vi "Set Conditional Symbols.vi"(0 "Project Path":path, 1 "w_niscope":bool, 2 "w_visa":bool, 11 "error in (no error)":errorcluster) -> (15 "error out":errorcluster)   [LabVIEW 2013]
doc: "VI sets conditional symbols in the project."
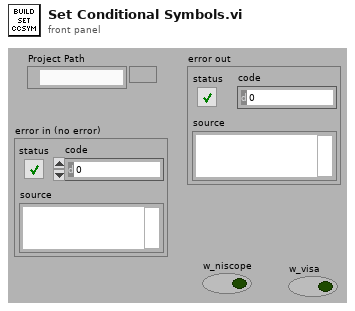
[diagram p1: front panel]
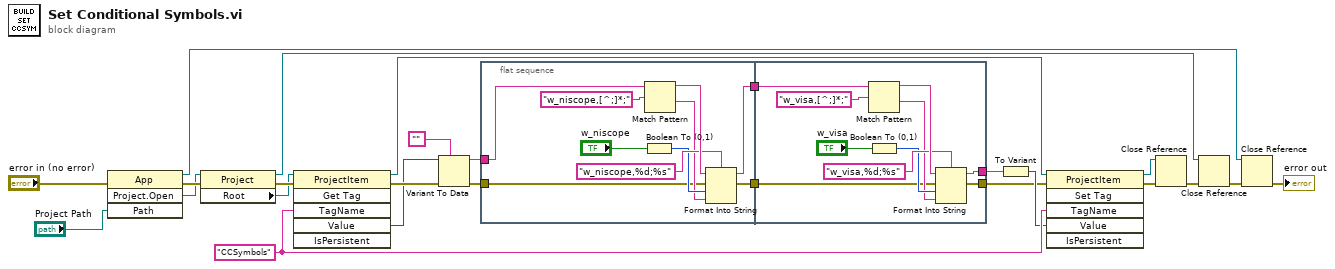
[diagram p0: block diagram]
diagram:
  w22 = "CCSymbols" ("Tag Name")
  n1 = invoke class="App" method="Project.Open"(error in="error in (no error)", "Path"="Project Path") -> (reference out=w13:refnum<vi>, error out=w14:errorcluster, "Project:Open"=w11:refnum<vi>)  [unwired: 2 in, 1 out]
  n2 = property class="Project"(reference=w11, error in=w14) -> (reference out=w12:refnum<vi>, error out=w21:errorcluster, "Root"=w2:refnum<vi>)
  n3 = invoke class="ProjectItem" method="Get Tag"(reference=w2, error in=w21, "TagName"=w22) -> (reference out=w1:refnum<vi>, error out=w24:errorcluster, "Value"=w23:variant)  [unwired: 3 in, 3 out]
  n4 = Variant To Data(error in=w24, type="", Variant=w23) -> (data=w10:string, error out=w9:errorcluster)
  n5 = flat-sequence {
    tunnel: w10 -> [w35]
    tunnel: w9 -> [w26]
    tunnel: [w28] -> w8
    tunnel: [w27] -> w7
    tunnel: w8 -> [w37]
    tunnel: w7 -> [w36]
    tunnel: [w39] -> w6
    tunnel: [w38] -> w4
    frame #0 {
      n6 = Boolean To (0,1)(Boolean="w_niscope") -> (0, 1=w30:i16)
      n7 = Match Pattern(string=w35, regular expression="w_niscope,[^;]*;") -> (before substring=w33:string, after substring=w29:string)  [unwired: 1 in, 2 out]
      n8 = Format Into String(format string="w_niscope,%d;%s", initial string=w33, error in=w26, w30, w29) -> (resulting string=w27:string, error out=w28:errorcluster)
    }
    frame #1 {
      n9 = Match Pattern(string=w36, regular expression="w_visa,[^;]*;") -> (before substring=w44:string, after substring=w40:string)  [unwired: 1 in, 2 out]
      n10 = Boolean To (0,1)(Boolean="w_visa") -> (0, 1=w41:i16)
      n11 = Format Into String(format string="w_visa,%d;%s", initial string=w44, error in=w37, w41, w40) -> (resulting string=w39:string, error out=w38:errorcluster)
    }
  }
  n12 = To Variant(anything=w6) -> (Variant=w5:variant)
  n13 = invoke class="ProjectItem" method="Set Tag"(reference=w1, error in=w4, "TagName"=w22, "Value"=w5) -> (reference out=w18:refnum<vi>, error out=w17:errorcluster)  [unwired: 2 in, 4 out]
  n14 = Close Reference(reference=w18, error in (no error)=w17) -> (error out=w15:errorcluster)
  n15 = Close Reference(reference=w12, error in (no error)=w15) -> (error out=w16:errorcluster)
  n16 = Close Reference(reference=w13, error in (no error)=w16) -> (error out=→"error out":errorcluster)
